vi "JoystickToDial.vi"(7 "Reset":bool, 9 "Reverse":bool, 10 "Y":dbl, 11 "X":dbl) -> (2 "Throttle":dbl(slide) scale=-1.0..1.0, 3 "Heading":dbl(knob) scale=-360.0..360.0)   [LabVIEW 2016]
panel:
  in  "Degree Snap":dbl=360.0
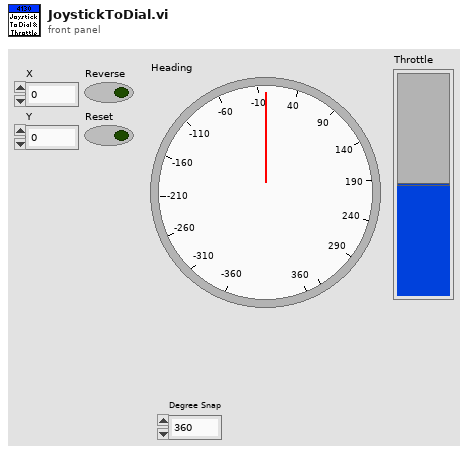
[diagram p1: front panel]
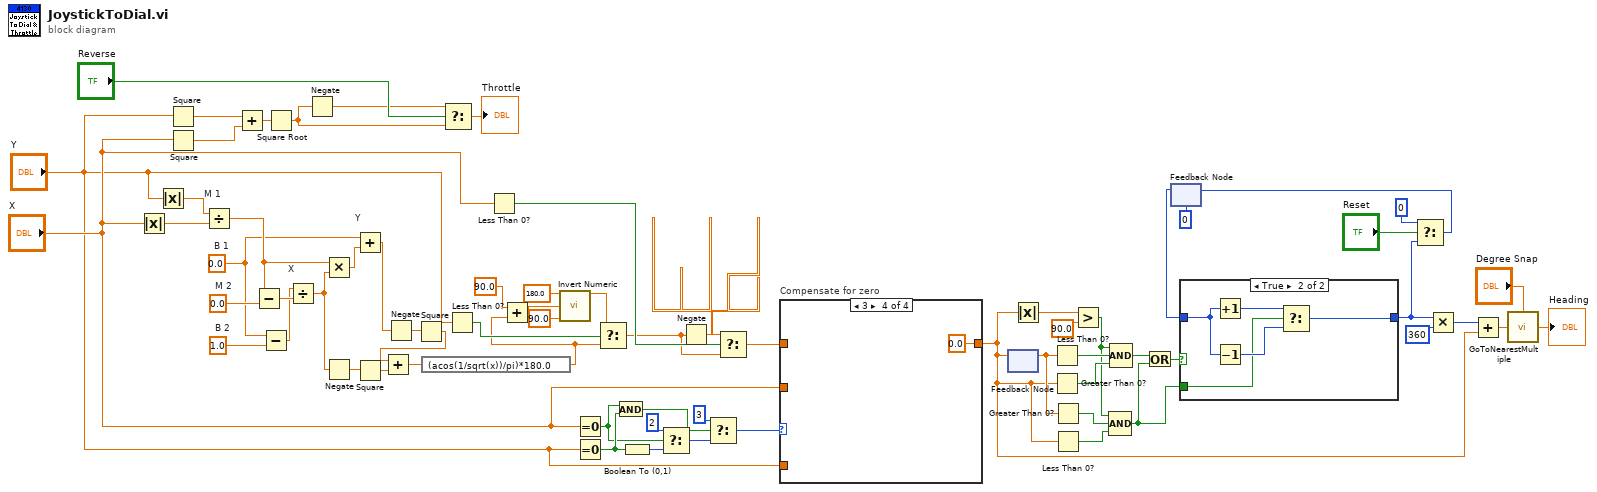
[diagram p0: block diagram]
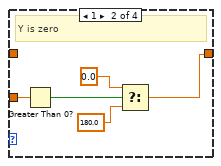
[diagram p3: hidden frame]
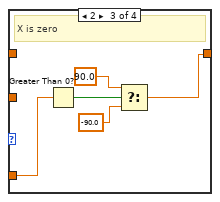
[diagram p4: hidden frame]
diagram:
  w66 = 0.0  # M 2
  w67 = 1.0  # B 2
  w55 = 0.0  # B 1
  n1 = Absolute Value(x="X") -> (abs(x)=w56:dbl)
  n2 = Absolute Value(x="Y") -> (abs(x)=w57:dbl)
  n3 = Square(x="Y") -> (x^2=w29:dbl)
  n4 = Square(x="X") -> (x^2=w28:dbl)
  n5 = Divide "M 1"(x=w57, y=w56) -> (x/y=w65:dbl)
  n6 = Add(x=w29, y=w28) -> (x+y=w27:dbl)
  n7 = Subtract(x=w65, y=w66) -> (x-y=w63:dbl)
  n8 = Subtract(x=w55, y=w67) -> (x-y=w62:dbl)
  n9 = Square Root(x=w27) -> (sqrt(x)=w26:dbl)
  n10 = Divide "X"(x=w62, y=w63) -> (x/y=w45:dbl)
  n11 = Negate(x=w26) -> (-x=w13:dbl)
  n12 = Multiply(x=w65, y=w45) -> (x*y=w64:dbl)
  n13 = Negate(x=w45) -> (-x=w61:dbl)
  n14 = Add "Y"(x=w55, y=w64) -> (x+y=w24:dbl)
  n15 = Square(x=w61) -> (x^2=w59:dbl)
  n16 = Negate(x=w24) -> (-x=w18:dbl)
  n17 = Square(x=w18) -> (x^2=w60:dbl)
  n18 = Add(x=w60, y=w59) -> (x+y=w58:dbl)
  n19 = expression code="(acos(1/sqrt(x))/pi)*180.0"(w58) -> (w51:dbl)
  n20 = Select(t=w13, s="Reverse", f=w26) -> (s? t:f=→"Throttle":dbl)
  n21 = Less Than 0?(x="Y") -> (x < 0?=w54:bool)
  n22 = Less Than 0?(x="X") -> (x < 0?=w52:bool)
  n23 = Add(x=90.0, y=w51) -> (x+y=w48:dbl)
  n24 = call "Invert Numeric.vi"("celing"=180.0, "Numeric"=w48, "floor"=90.0) -> ("coerced(Inverted)"=w17:dbl)  [unwired: 10 in, 2 out]
  n25 = Equal To 0?(x="X") -> (x = 0?=w4:bool)
  n26 = Equal To 0?(x="Y") -> (x = 0?=w5:bool)
  n27 = Select(t=w17, s=w54, f=w51) -> (s? t:f=w47:dbl)
  n28 = And(x=w4, y=w5) -> (x .and. y?=w3:bool)
  n29 = Boolean To (0,1)(Boolean=w5) -> (0, 1=w10:i16)
  n30 = Select(t=i16 2, s=w4, f=w10) -> (s? t:f=w8:i16)
  n31 = Negate(x=w47) -> (-x=w46:dbl)
  n32 = Select(t=i16 3, s=w3, f=w8) -> (s? t:f=w6:i16)
  n33 = Select(t=w46, s=w52, f=w47) -> (s? t:f=w12:dbl)
  n34 = case "Compensate for zero" shown="3" w6 {
    tunnel: w12 -> [w68 _ _ _]
    tunnel: [w68 w69 w75 0.0 ("f")] -> w11
    tunnel: "X" -> [_ w73 _ _]
    tunnel: "Y" -> [_ _ w74 _]
    frame 0, Default {
    }
    frame 1 {
      # "Y is zero"
      n35 = Greater Than 0?(x=w73) -> (x > 0?=w72:bool)
      n36 = Select(t=0.0, s=w72, f=180.0) -> (s? t:f=w69:dbl)
    }
    frame 2 {
      # "X is zero"
      n37 = Greater Than 0?(x=w74) -> (x > 0?=w78:bool)
      n38 = Select(t=90.0, s=w78, f=-90.0) -> (s? t:f=w75:dbl)
    }
    frame 3 {
    }
  }
  n39 = feedback #1() -> (w36:dbl)  [unwired: 1 in]
  n40 = feedback-in #1(w11) -> ()
  n41 = Absolute Value(x=w11) -> (abs(x)=w39:dbl)
  n42 = Less Than 0?(x=w36) -> (x < 0?=w38:bool)
  n43 = Greater Than 0?(x=w11) -> (x > 0?=w37:bool)
  n44 = Greater Than 0?(x=w36) -> (x > 0?=w34:bool)
  n45 = Less Than 0?(x=w11) -> (x < 0?=w33:bool)
  n46 = Greater?(x=w39, y=90.0) -> (0:w35:bool)
  n47 = Compound Arithmetic op=AND(w35, w34, w33) -> (w30:bool)
  n48 = Compound Arithmetic op=AND(w35, w38, w37) -> (w31:bool)
  n49 = Or(x=w31, y=w30) -> (x .or. y?=w32:bool)
  n50 = feedback #2(0) -> (w44:i32)
  n51 = case shown="True" w32 {
    tunnel: [w80 w83] -> w22
    tunnel: w44 -> [w80 w82]
    tunnel: w30 -> [_ w81]
    frame False {
    }
    frame True {
      n52 = Increment(x=w82) -> (x+1=w84:i32)
      n53 = Decrement(x=w82) -> (x-1=w85:i32)
      n54 = Select(t=w84, s=w81, f=w85) -> (s? t:f=w83:i32)
    }
  }
  n55 = Select(t=0, s="Reset", f=w22) -> (s? t:f=w21:i32)
  n56 = feedback-in #2(w21) -> ()
  n57 = Multiply(x=w22, y=360) -> (x*y=w41:i32)
  n58 = Add(x=w41, y=w11) -> (x+y=w16:dbl)
  n59 = call "GoToNearestMultiple.vi"("Multiple"="Degree Snap", "Numeric"=w16) -> ("Snapped Numeric"=→"Heading":dbl)  [unwired: 13 in]
